vi "Create Notifiers.vi"(8 "error in (no error)":errorcluster) -> (0 "error out":errorcluster, 2 "ques":cluster{"logging que":refnum<queue>}, 3 "notifiers cluster":T1)   [LabVIEW 2020]
uses:
  _controls/Notifiers.ctl
  _controls/Logging Cluster.ctl
  _controls/Exp Params.ctl
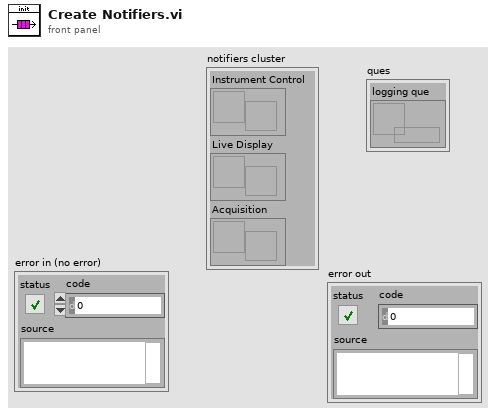
[diagram p1: front panel]
types:
  T1 = typedef "Notifiers.ctl" = cluster{"Instrument Control":refnum<notifier>, "Live Display":refnum<notifier>, "Acquisition":refnum<notifier>}
  T2 = typedef "Logging Cluster.ctl" = cluster{"Image Data Array":u8[], "Buffer Number":i32, "Timestamp (um)":u64, "Exp params":T3}
  T3 = typedef "Exp Params.ctl" = cluster{"Experiment Type":string, "Experiment Name":string, "ExpPath":path, "Save As":string, "TSFrames":i32, "TSfps":dbl, "Streaming":bool, "tdms ref":refnum<k34>, "frame #":i64, "Full Path":path, "PeakOnQueue":bool}
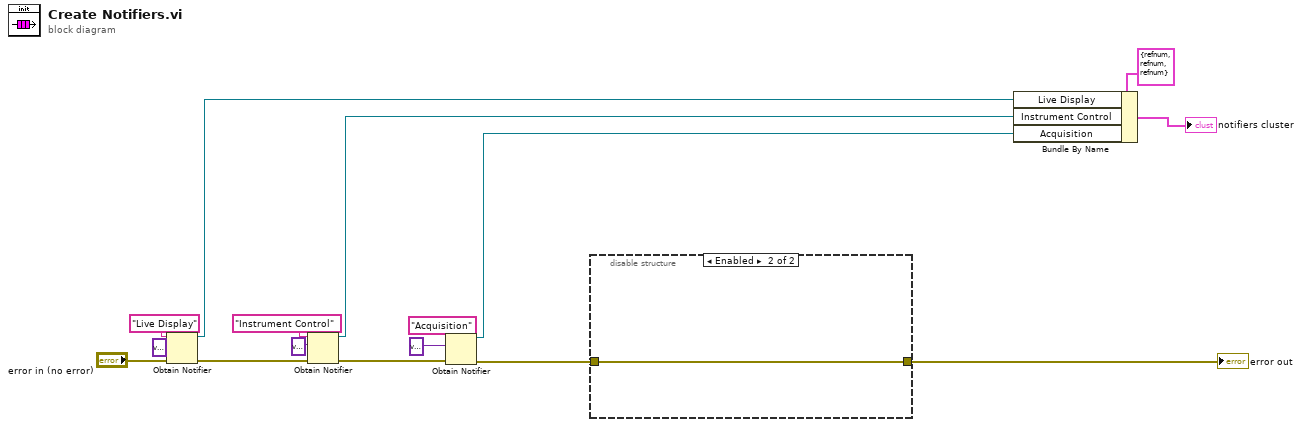
[diagram p0: block diagram]
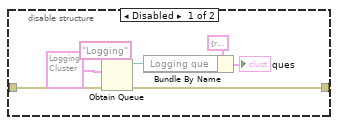
[diagram p2: hidden frame]
diagram:
  n1 = Obtain Notifier(name (unnamed)="Live Display", notification data type=variant, error in (no error)="error in (no error)") -> (notifier out=w6:refnum<notifier>, error out=w14:errorcluster)  [unwired: 1 in, 1 out]
  n2 = Obtain Notifier(name (unnamed)="Instrument Control", notification data type=variant, error in (no error)=w14) -> (notifier out=w5:refnum<notifier>, error out=w8:errorcluster)  [unwired: 1 in, 1 out]
  n3 = Obtain Notifier(name (unnamed)="Acquisition", notification data type=variant, error in (no error)=w8) -> (notifier out=w4:refnum<notifier>, error out=w2:errorcluster)  [unwired: 1 in, 1 out]
  n4 = disable-structure shown="Enabled" {
    disable-tunnel: w2 -> [w18 w24]
    disable-tunnel: [w17 w24] -> w1
    frame Disabled {
      n5 = Obtain Queue(name (unnamed)="Logging", element data type=T2 {"Image Data Array"=[], "Buffer Number"=0, "Timestamp (um)"=0, "Exp params"={"Experiment Type"="", "Experiment Name"="Experiment_1", "ExpPath"=path "D:/Data", "Save As"="TIFF", "TSFrames"=1000, "TSfps"=1.0, "Streaming"=FALSE, "tdms ref"=refnum, "frame #"=0, "Full Path"=path "", "PeakOnQueue"=FALSE}}, error in (no error)=w18) -> (queue out=w21:refnum<queue>, error out=w17:errorcluster)  [unwired: 2 in, 1 out]
      n6 = Bundle By Name(cluster=cluster{"Logging que":refnum<queue>} {"Logging que"=refnum} ("output cluster"), "Logging que"=w21) -> (→"ques":cluster{"Logging que":refnum<queue>})
    }
    frame Enabled {
    }
  }
  "error out" <- w1
  n7 = Bundle By Name(cluster=T1 {"Instrument Control"=refnum, "Live Display"=refnum, "Acquisition"=refnum} ("notifiers cluster"), "Live Display"=w6, "Instrument Control"=w5, "Acquisition"=w4) -> (→"notifiers cluster":T1)
